vi "Close Ref.vi"(8 "error in (no error)":errorcluster, 11 "ARS-0220 in":refnum<class "ARS-0220.lvclass">) -> (0 "error out":errorcluster, 3 "ARS-0220 out":refnum<class "ARS-0220.lvclass">)   [LabVIEW 2016, in "Environment Chamber.lvlib" / "ARS-0220.lvclass"]
uses:
  ARS-0220.lvclass
  ARS-0220.lvclass/ARS-0220.ctl
  Support Libraries/Climatic Chamber/Climatic Chamber.lvlib
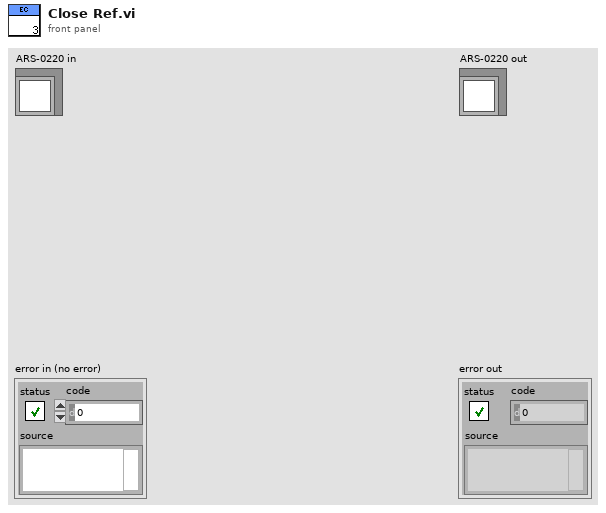
[diagram p1: front panel]
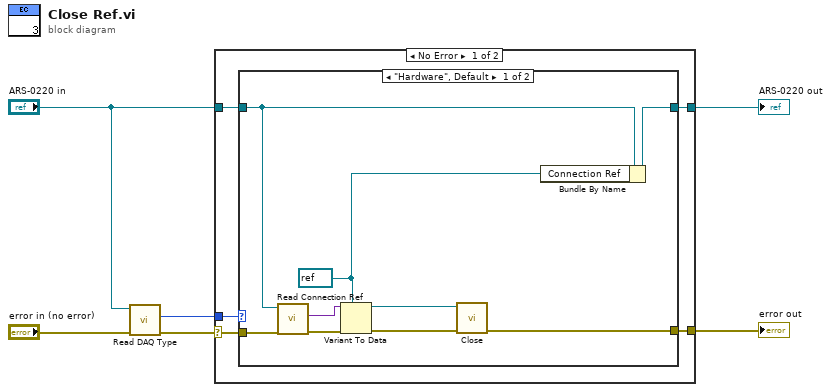
[diagram p0: block diagram]
diagram:
  n1 = call "Read DAQ Type.vi"("error in (no error)"="error in (no error)", "ARS-0220 in"="ARS-0220 in") -> ("error out"=w5:errorcluster, "DAQ Type"=w3:enum16{"Hardware", "Simulation"})  [unwired: 7 in, 1 out]
  n2 = case shown="No Error" w5 {
    selector: w5 -> [w9 w23]
    tunnel: "ARS-0220 in" -> [w10 w24]
    tunnel: w3 -> [w11 _]
    tunnel: [w8 w24] -> w2
    tunnel: [w7 w23] -> w1
    frame No Error {
      n3 = case shown="\"Hardware\", Default" w11 {
        tunnel: w10 -> [w15 w22]
        tunnel: w9 -> [w20 w21]
        tunnel: [w13 w22] -> w8
        tunnel: [w14 w21] -> w7
        frame "Hardware", Default {
          w12 = refnum<visa-resource-name> refnum ("VISA resource name")
          n4 = call "Read Connection Ref.vi"("error in (no error)"=w20, "ARS-0220 in"=w15) -> ("error out"=w19:errorcluster, "Connection Ref"=w18:variant)  [unwired: 7 in, 1 out]
          n5 = Variant To Data(error in=w19, type=w12, Variant=w18) -> (data=w16:refnum<visa-resource-name>, error out=w17:errorcluster)
          n6 = call "Close.vi"("error in (no error)"=w17, "VISA resource name"=w16) -> ("error out"=w14:errorcluster)  [unwired: 9 in]
          n7 = Bundle By Name(cluster=w15, "Connection Ref"=w12) -> (w13:refnum<class "ARS-0220.lvclass">)
        }
        frame "Simulation" {
        }
      }
    }
    frame Error {
    }
  }
  "error out" <- w1
  "ARS-0220 out" <- w2
